vi "Set Serial Communicator.vi"(10 "SerialProtocols.lvlib:SerialCommunicator.lvclass":refnum<class "SerialCommunicator.lvclass">, 11 "Tovey9150 in":refnum<class "Tovey 9150.lvclass">) -> (3 "Tovey9150 out":refnum<class "Tovey 9150.lvclass">)   [LabVIEW 2015, in "Tovey 9150.lvclass"]
uses:
  Tovey 9150.lvclass
  <userlib>/Common/SerialProtocols/SerialCommunicator/SerialCommunicator.lvclass
  Tovey 9150.lvclass/Tovey 9150.ctl
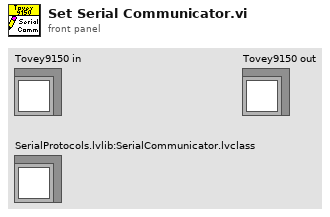
[diagram p1: front panel]
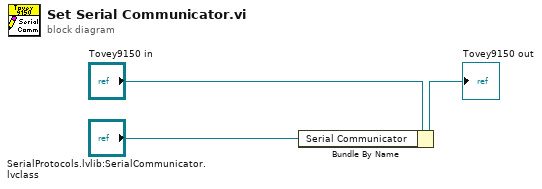
[diagram p0: block diagram]
diagram:
  n1 = Bundle By Name(cluster="Tovey9150 in", "Serial Communicator"="SerialProtocols.lvlib:SerialCommunicator.lvclass") -> (→"Tovey9150 out":refnum<class "Tovey 9150.lvclass">)
